vi "Get Strings from Ref.vi"(8 "error in (no error)":errorcluster, 9 "Label Prefix":string, 10 "GObj Refnum in":refnum<vi>, 11 "RingControl in":refnum<class "RingControl.lvclass">) -> (0 "error out":errorcluster, 1 "Valid?":bool, 2 "GObj Refnum out":refnum<vi>, 3 "RingControl out":refnum<class "RingControl.lvclass">, 4 "GObj Name":string)   [LabVIEW 2013, in "SET Project Data.lvlib" / "RingControl.lvclass"]
uses:
  RingControl.lvclass
  Control/Control.lvclass
  GObject/GObject.lvclass/GObject.ctl
  GObject/Write UID.vi
  SET Project Data.lvlib
  GObject/GObject.lvclass
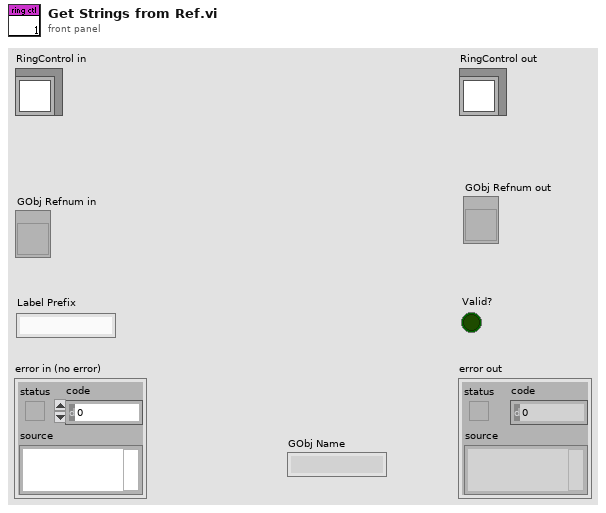
[diagram p1: front panel]
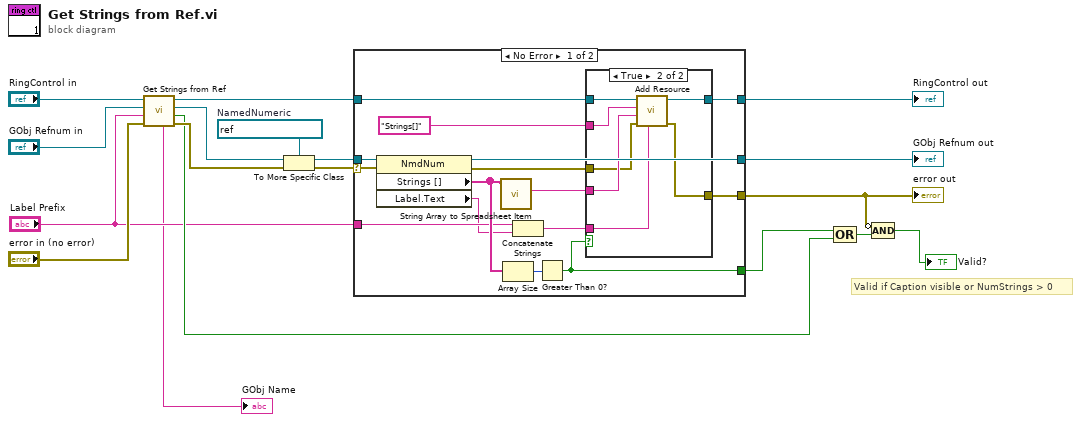
[diagram p0: block diagram]
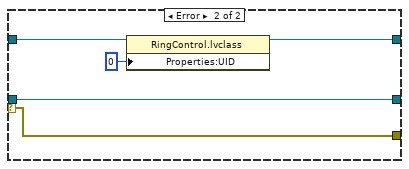
[diagram p3: hidden frame]
diagram:
  w13 = refnum<vi> refnum  # NamedNumeric
  # "Valid if Caption visible or NumStrings > 0"
  n1 = call-parent "Get Strings from Ref.vi"("error in (no error)"="error in (no error)", "Label Prefix"="Label Prefix", "GObj Refnum in"="GObj Refnum in", "Control in"="RingControl in") -> ("error out"=w14:errorcluster, "Valid?"=w6:bool, "GObj Refnum out"=w15:refnum<vi>, "Control out"=w10:refnum<class "RingControl.lvclass">, "GObj Name"=→"GObj Name":string)  [unwired: 3 in]
  n2 = To More Specific Class(target class=w13, reference=w15, error in=w14) -> (specific class reference=w12:refnum<vi>, error out=w11:errorcluster)
  n3 = case shown="No Error" w11 {
    selector: w11 -> [w32 w46]
    tunnel: w12 -> [w33 w47]
    tunnel: w10 -> [w28 w45]
    tunnel: [w27 w43] -> w9
    tunnel: [w20 w46] -> w4
    tunnel: [w31 w47] -> w8
    tunnel: [w19 _] -> w7
    tunnel: "Label Prefix" -> [w26 _]
    frame No Error {
      n4 = property class="NmdNum"(reference=w33, error in=w32) -> (reference out=w31:refnum<vi>, error out=w21:errorcluster, "Strings []"=w29:string[], "Label.Text"=w25:string)
      n5 = call "String Array to Spreadsheet Item.vi"("Strings [] (ASCII)"=w29) -> ("Spreadsheet Item (ASCII)"=w23:string)  [unwired: 10 in]
      n6 = Array Size(array=w29) -> (size(s)=w30:i32)
      n7 = Concatenate Strings(w26, w25) -> (w24:string)
      n8 = Greater Than 0?(x=w30) -> (x > 0?=w19:bool)
      n9 = case shown="True" w19 {
        tunnel: w28 -> [w35 w42]
        tunnel: [w35 w41] -> w27
        tunnel: w24 -> [_ w40]
        tunnel: w23 -> [_ w39]
        tunnel: "Strings[]" -> [_ w38]
        tunnel: w21 -> [w34 w37]
        tunnel: [w34 w36] -> w20
        frame False {
        }
        frame True {
          n10 = call "Add Resource.vi"("TagPrefix"=w40, "error in (no error)"=w37, "ItemText"=w39, "ItemName"=w38, "GObject in"=w42) -> ("error out"=w36:errorcluster, "GObject out"=w41:refnum<class "RingControl.lvclass">)  [unwired: 5 in]
        }
      }
    }
    frame Error {
      n11 = property class="RingControl.lvclass"(reference=w45, "Properties:UID"=0 ("UID")) -> (reference out=w43:refnum<class "RingControl.lvclass">)  [unwired: 1 in, 1 out]
    }
  }
  "error out" <- w4
  "RingControl out" <- w9
  "GObj Refnum out" <- w8
  n12 = Compound Arithmetic op=OR(w7, w6) -> (w5:bool)
  n13 = Compound Arithmetic op=AND(invert w4, w5) -> (→"Valid?":bool)
